vi "Write Connection Information.vi"(8 "error in (no error)":errorcluster, 10 "Connection Information":path, 11 "ADODB in":refnum<class "ADODB.lvclass">) -> (0 "error out":errorcluster, 3 "ADODB out":refnum<class "ADODB.lvclass">)   [LabVIEW 2020, in "ADODB.lvclass"]
uses:
  ADODB.lvclass
  ADODB.lvclass/ADODB.ctl
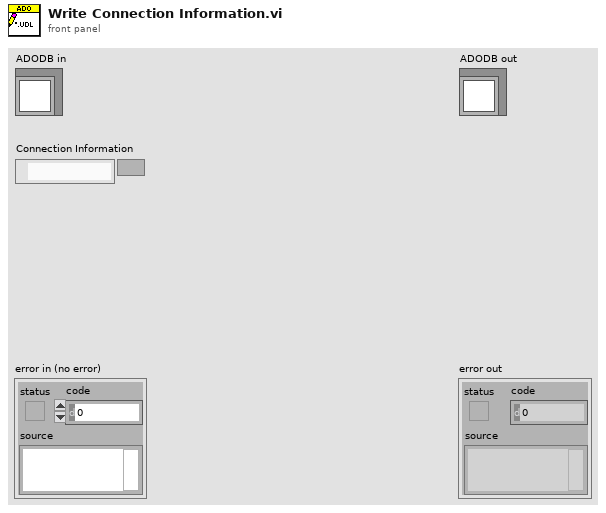
[diagram p1: front panel]
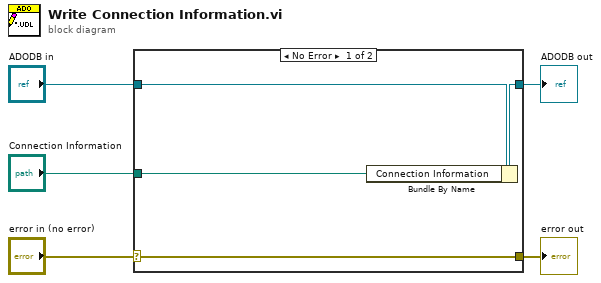
[diagram p0: block diagram]
diagram:
  n1 = case shown="No Error" "error in (no error)" {
    selector: "error in (no error)" -> [w9 w10]
    tunnel: [w9 w10] -> w4
    tunnel: [w7 w11] -> w2
    tunnel: "ADODB in" -> [w8 w11]
    tunnel: "Connection Information" -> [w6 _]
    frame No Error {
      n2 = Bundle By Name(cluster=w8, "Connection Information"=w6) -> (w7:refnum<class "ADODB.lvclass">)
    }
    frame Error {
    }
  }
  "error out" <- w4
  "ADODB out" <- w2
